vi "tlc_Record Dialog Box.vi"(8 "error in (no error)":errorcluster) -> (0 "error out":errorcluster, 2 "Output Cue":T1 {"Channels"."Intensity" min=0.0 max=100.0 step=1.0 format="%#.0f"}, 3 "Cancelled?":bool)   [LabVIEW 2009]
doc: "Use this template to create a dialog box with event handling."
uses:
  Controls/tlc_Cue_Information.ctl
  Controls/channel.ctl
  Modules/Cue/tlc_Cue_Information Command.ctl
panel:
  in  "Cue Information":T1={"Cue Name"="", "Wait Time (s)"=0, "Fade Time (s)"=1, "Follow Time (s)"=0, "Channels"=[]} {"Channels"."Intensity" min=0.0 max=100.0 step=1.0 format="%#.0f"; "Fade Time (s)" min=1}
  in  "Cancel":bool
  in  "OK":bool
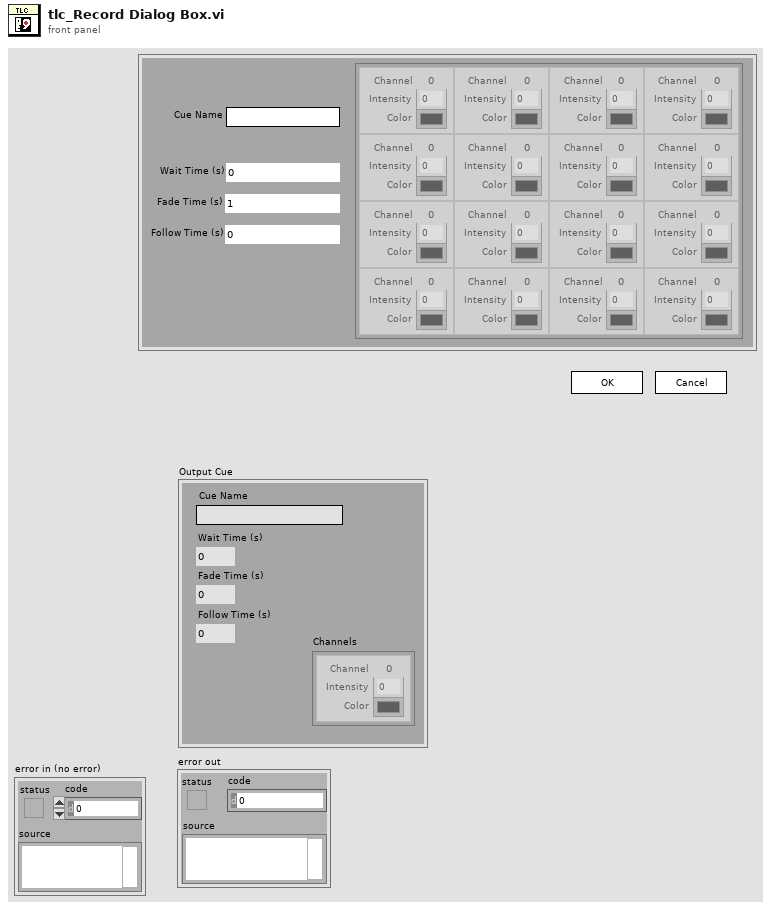
[diagram p1: front panel]
types:
  T1 = typedef "tlc_Cue_Information.ctl" = cluster{"Cue Name":string, "Wait Time (s)":u32, "Fade Time (s)":u32, "Follow Time (s)":u32, "Channels":T2[][]}
  T2 = typedef "channel.ctl" = cluster{"Intensity":dbl, " Color":u32, "Channel":i32}
  T3 = typedef "tlc_Cue_Information Command.ctl" = enum16{"Add Cue", "Get Cue Values", "Set Cue Values", "Get Number of Cues", "Initialize", "Get Empty Cue"}
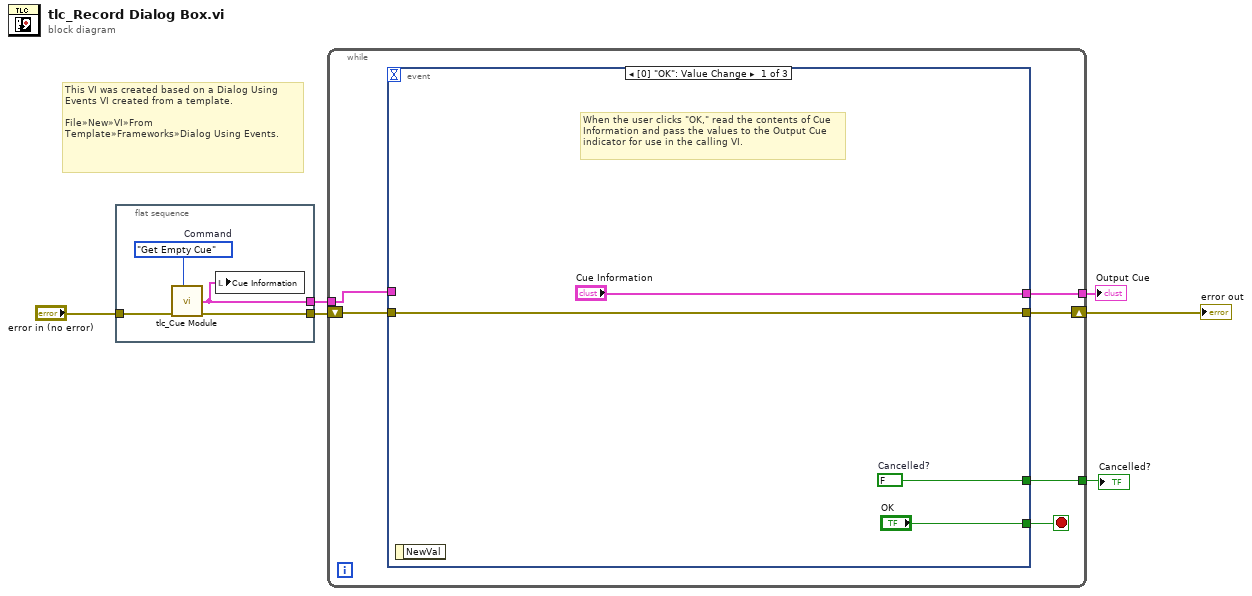
[diagram p0: block diagram]
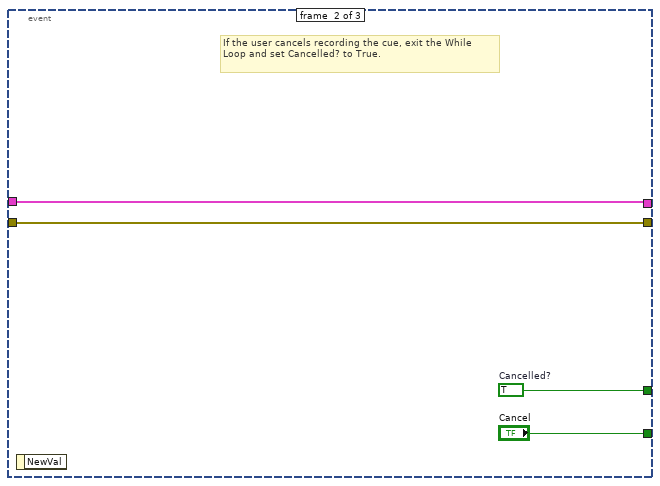
[diagram p2: hidden frame]
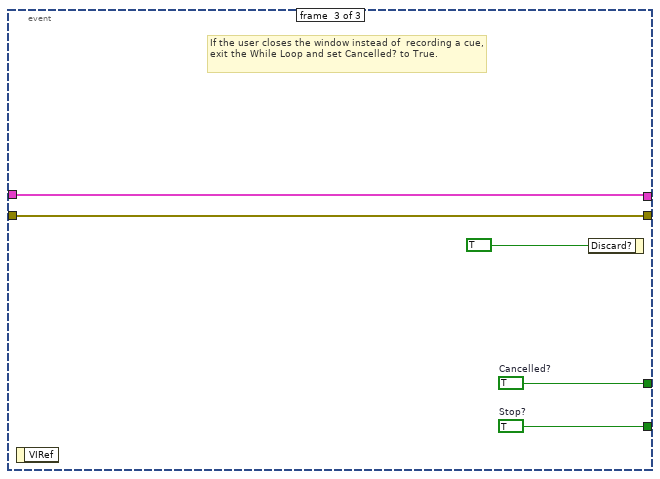
[diagram p3: hidden frame]
diagram:
  # "This VI was created based on a Dialog Using Events VI created from a template.   \n\nFile»New»VI»From Template»Frameworks»Dialog Using Events."
  n1 = flat-sequence {
    tunnel: [w10] -> w5
    tunnel: [w9] -> w4
    tunnel: "error in (no error)" -> [w8]
    frame #0 {
      w7 = tlc_Cue_Information_Command."Get Empty Cue"  # Command
      n2 = call "tlc_Cue Module.vi"("Command"=w7, "error in (no error)"=w8) -> ("error out"=w10:errorcluster, "Cue Output"=w9:T1)  [unwired: 6 in, 1 out]
      n3 = local write "Cue Information"(w9) -> ()
    }
  }
  n4 = while {
    tunnel: [w15] -> w6
    tunnel: [w14] -> w1
    shift-right: [w12] -> w2
    shift-left: w5 -> [w11]
    tunnel: w4 -> [w13]
    stop <- w16 stop-if-true
    n5 = event shown="[0] \"OK\": Value Change" {
      selector: _ -> [_ _ _]
      dyn-events: _ -> [_ _ _]
      timeout: _ -> [_ _ _]
      tunnel: ["OK" "Cancel" w28] -> w16
      tunnel: [w20 w24 w27] -> w15
      tunnel: ["Cue Information" w22 w26] -> w14
      tunnel: w13 -> [_ w22 w26]
      tunnel: [w17 w21 w25] -> w12
      tunnel: w11 -> [w17 w21 w25]
      event #0 {
        w20 = FALSE  # Cancelled?
        # "When the user clicks \"OK,\" read the contents of Cue Information and pass the values to the Output Cue indicator for use in the calling VI."
        n6 = event-data() -> ()  [unwired: 1 in, 1 out]
      }
      event #1 {
        w24 = TRUE  # Cancelled?
        # "If the user cancels recording the cue, exit the While Loop and set Cancelled? to True."
        n7 = event-data() -> ()  [unwired: 1 in, 1 out]
      }
      event #2 {
        w27 = TRUE  # Cancelled?
        w28 = TRUE  # Stop?
        # "If the user closes the window instead of  recording a cue, exit the While Loop and set Cancelled? to True."
        n8 = event-data() -> ()  [unwired: 1 in, 1 out]
        n9 = event-data("Discard?"=TRUE) -> ()  [unwired: 1 in, 1 out]
      }
    }
  }
  "Cancelled?" <- w6
  "error out" <- w2
  "Output Cue" <- w1
